vi "stream_only_test.vi"() -> ()   [LabVIEW 2025, in "LabJackEKG.lvlib"]
uses:
  LabJackEKG.lvlib
  <vilib>/Analysis/NI_AALPro.lvlib
panel:
  in  "Sampling Frequency [Hz]":dbl=2500.0
  out "stop":bool
  in  "Samples":i64
  in  "Window":bool
  in  "milliseconds to wait":u32=100
  out "size(s)":i32
  out "Waveform Chart":cluster{dbl, dbl}(graph)
  in  "Number of Stickers":i64
  in  "Samping Window [s]":dbl
  out "error out":errorcluster
  in  "stop":bool
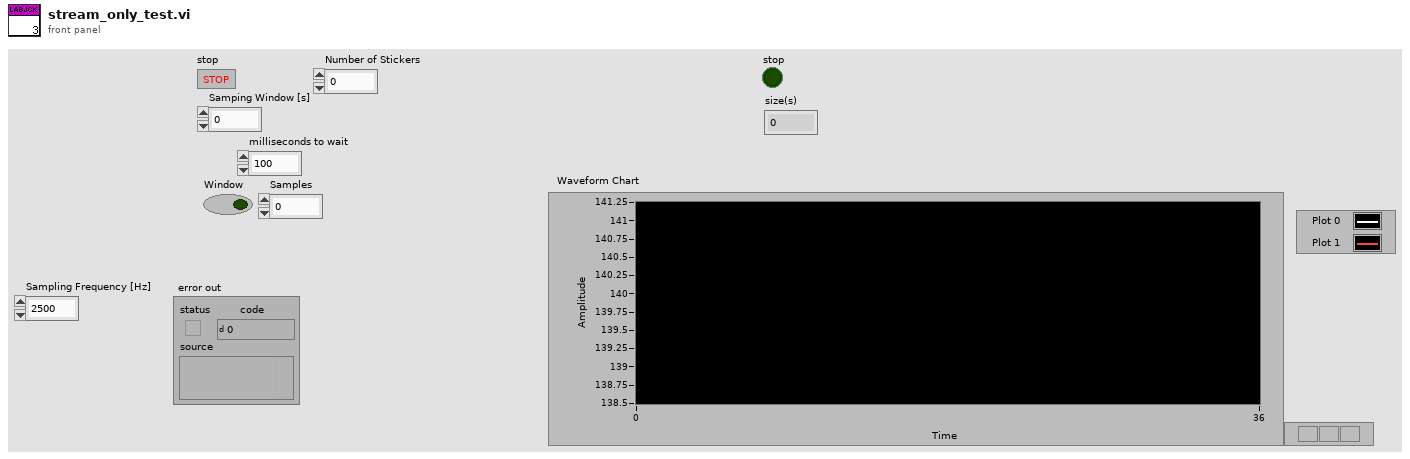
[diagram p1: front panel]
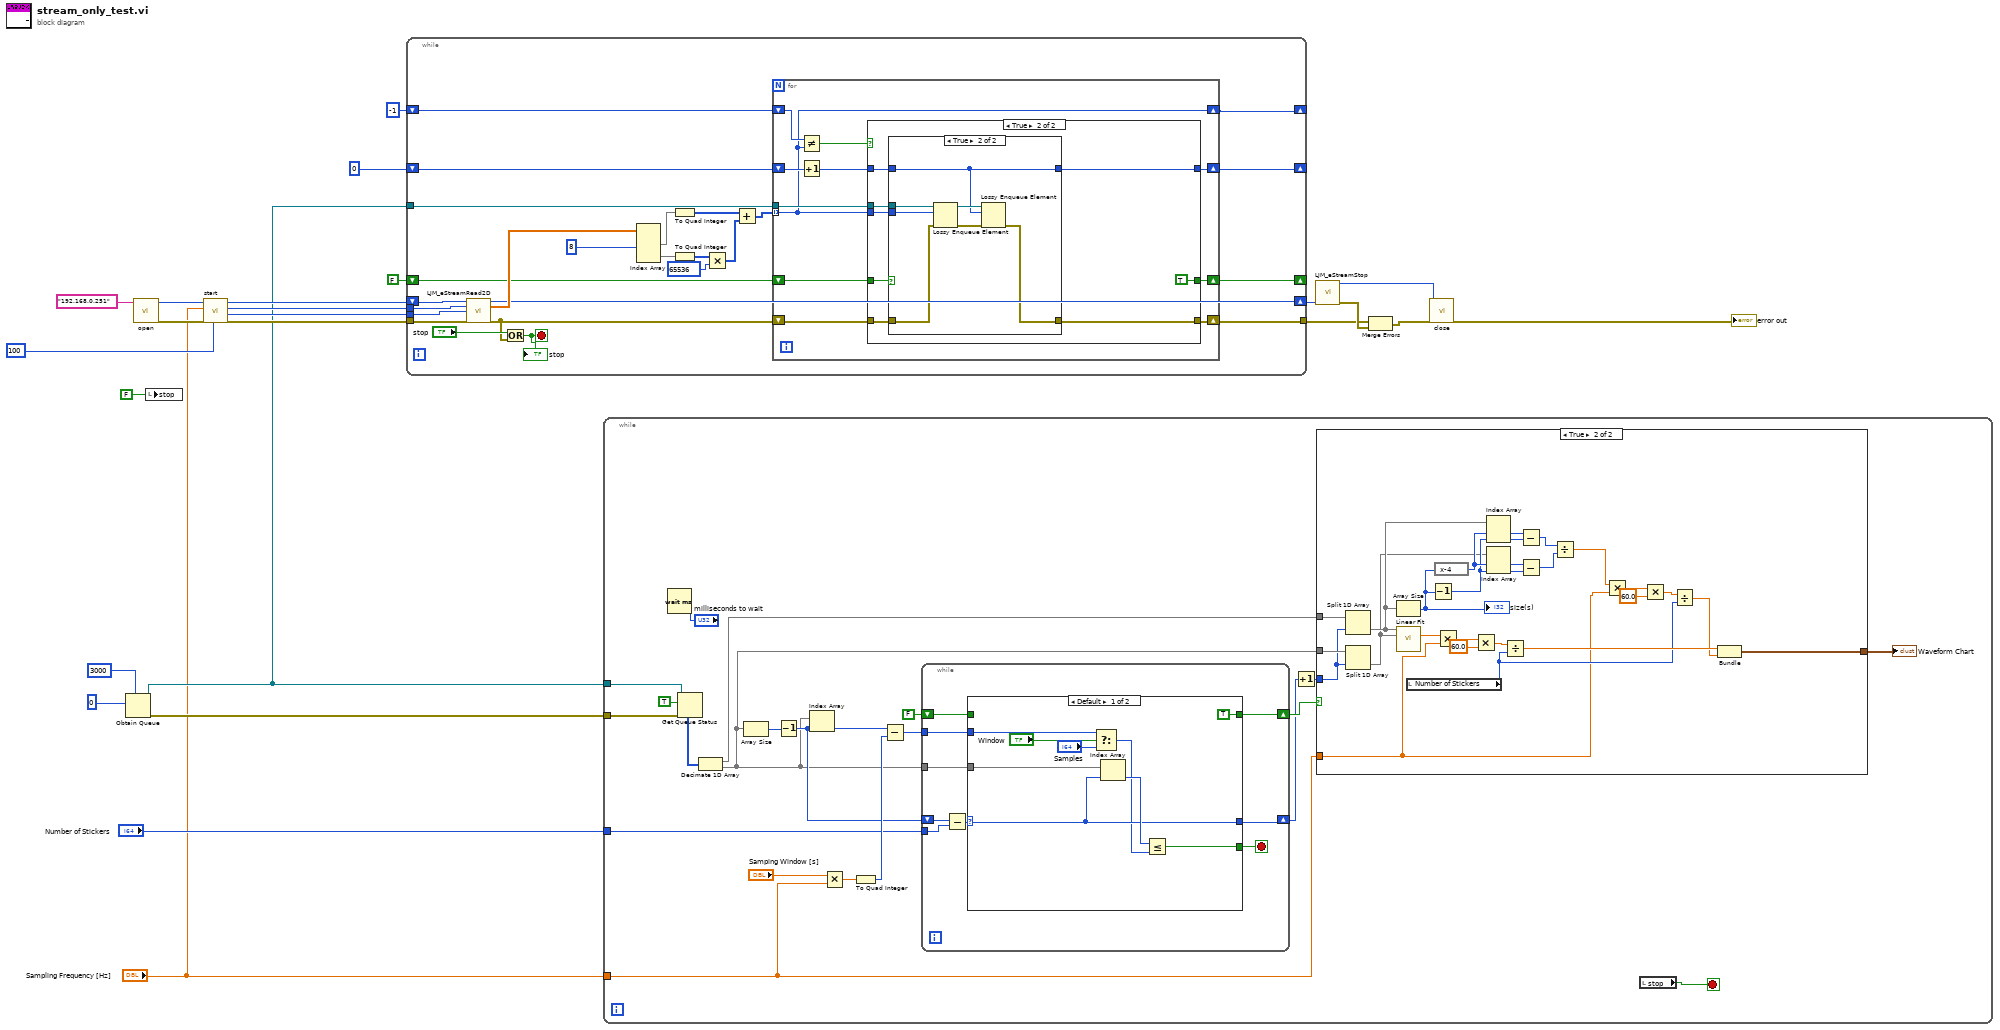
[diagram p0: block diagram]
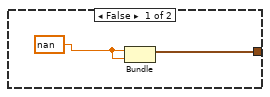
[diagram p4: hidden frame]
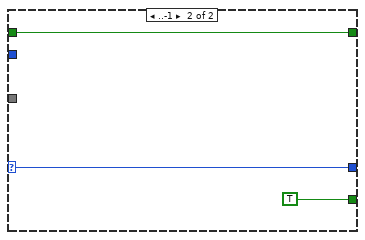
[diagram p5: hidden frame]
diagram:
  n1 = Obtain Queue(max queue size (-1, unlimited)=3000, element data type=i64 0) -> (queue out=w12:refnum<queue>, error out=w14:errorcluster)  [unwired: 3 in, 1 out]
  n2 = call "open.vi"("IP Address (LJM_idANY )"="192.168.0.251") -> ("error out"=w24:errorcluster, "Handle"=w23:i32)  [unwired: 8 in, 1 out]
  n3 = local write "stop"(FALSE ("x .or. y?")) -> ()
  n4 = call "start.vi"("Period [ms]"=100, "error in (no error)"=w24, "Scan Rate (Hz)"="Sampling Frequency [Hz]", "Handle In"=w23) -> ("error out"=w22:errorcluster, "NumReadAddresses"=w19:i32, "ScansPerRead Out"=w20:i32, "Handle Out"=w21:i32)  [unwired: 4 in]
  n5 = while {
    tunnel: w22 -> [w49]
    tunnel: [w38] -> w3
    tunnel: w20 -> [w47]
    tunnel: w19 -> [w48]
    shift-right: [w43] -> w7
    shift-left: w21 -> [w46]
    tunnel: w12 -> [w40]
    shift-right: [w33] -> _
    shift-left: i64 -1 -> [w34]
    shift-right: [w36] -> _
    shift-left: i64 0 -> [w37]
    shift-right: [w25] -> _
    shift-left: FALSE ("x .or. y?") -> [w26]
    stop <- w32 stop-if-true
    n6 = call <vilib>:"LJM_eStreamRead2D.vi"("Handle In"=w46, "ScansPerRead"=w47, "NumAddresses"=w48, "error in"=w49) -> ("Handle Out"=w43:i32, "aData Out"=w45:dbl[][], "error out"=w39:errorcluster)  [unwired: 7 in, 2 out]
    n7 = Or(x="stop", y=w39) -> (x .or. y?=w32:bool)
    "stop" <- w32
    n8 = Index Array(array=w45, index (col) #1=8 ("disabled index (col)")) -> (element #1=w41:dbl[], element #2=w31:dbl[])  [unwired: 3 in]
    n9 = To Quad Integer(1:w41) -> (0:w35:i64[])
    n10 = To Quad Integer(1:w31) -> (0:w30:i64[])
    n11 = Multiply(x=w30, y=i64 65536 ("x")) -> (x*y=w27:i64[])
    n12 = Add(x=w35, y=w27) -> (x+y=w28:i64[])
    n13 = for {
      tunnel: w28 -> [w54] mode=indexing
      tunnel: w40 -> [w60]
      shift-right: [w59] -> w38
      shift-left: w39 -> [w58]
      shift-right: [w57] -> w36
      shift-left: w37 -> [w56]
      shift-right: [w54] -> w33
      shift-left: w34 -> [w55]
      shift-right: [w52] -> w25
      shift-left: w26 -> [w51]
      n14 = Not Equal?(x=w55, y=w54) -> (x != y?=w50:bool)
      n15 = Increment(x=w56) -> (x+1=w53:i64)
      n16 = case shown="True" w50 {
        tunnel: w60 -> [_ w71]
        tunnel: [w63 w68] -> w59
        tunnel: w58 -> [w63 w70]
        tunnel: w54 -> [_ w69]
        tunnel: [w62 w64] -> w57
        tunnel: w53 -> [w62 w67]
        tunnel: [w61 TRUE] -> w52
        tunnel: w51 -> [w61 w65]
        frame False {
        }
        frame True {
          n17 = case shown="True" w65 {
            tunnel: w71 -> [_ w80]
            tunnel: w70 -> [w73 w78]
            tunnel: w69 -> [_ w77]
            tunnel: [w73 w76] -> w68
            tunnel: w67 -> [w72 w74]
            tunnel: [w72 w74] -> w64
            frame False {
            }
            frame True {
              n18 = Lossy Enqueue Element(queue=w80, element=w77, error in (no error)=w78) -> (queue out=w75:refnum<queue>, error out=w79:errorcluster)  [unwired: 2 out]
              n19 = Lossy Enqueue Element(queue=w75, element=w74, error in (no error)=w79) -> (error out=w76:errorcluster)  [unwired: 3 out]
            }
          }
        }
      }
    }
  }
  n20 = while {
    tunnel: w12 -> [w102]
    tunnel: w14 -> [w101]
    tunnel: "Number of Stickers" -> [w94]
    tunnel: "Sampling Frequency [Hz]" -> [w83]
    stop <- w84 stop-if-true
    n21 = Wait (ms)(milliseconds to wait="milliseconds to wait") -> ()  [unwired: 1 out]
    n22 = Get Queue Status(queue=w102, return elements? (F)=TRUE, error in (no error)=w101) -> (elements=w100:i64[])  [unwired: 7 out]
    n23 = Decimate 1D Array(w100) -> (w89:i64[], w82:i64[])
    n24 = Array Size(array=w82) -> (size(s)=w91:i32)
    n25 = Decrement(x=w91) -> (x-1=w90:i32)
    n26 = Index Array(array=w82, index=w90) -> (element=w96:i64)
    n27 = Multiply(x="Samping Window [s]", y=w83) -> (x*y=w99:dbl)
    n28 = To Quad Integer(1:w99) -> (0:w97:i64)
    n29 = Subtract(x=w96, y=w97) -> (x-y=w95:i64)
    n30 = while {
      tunnel: w95 -> [w138]
      shift-right: [w135] -> w86
      shift-left: w90 -> [w132]
      tunnel: w94 -> [w140]
      tunnel: w82 -> [w134]
      shift-right: [w136] -> w88
      shift-left: FALSE -> [w133]
      stop <- w137 stop-if-true
      n31 = Subtract(x=w132, y=w140) -> (x-y=w139:i64)
      n32 = case shown="Default" w139 {
        selector: w139 -> [w145 w151]
        tunnel: w134 -> [w149 _]
        tunnel: w138 -> [w147 _]
        tunnel: [w146 TRUE] -> w137
        tunnel: [TRUE w150] -> w136
        tunnel: [w145 w151] -> w135
        tunnel: w133 -> [_ w150]
        frame Default {
          n33 = Select(t=w147, s="Window", f="Samples") -> (s? t:f=w143:i64)
          n34 = Index Array(array=w149, index=w145) -> (element=w148:i64)
          n35 = Less Or Equal?(x=w148, y=w143) -> (x <= y?=w146:bool)
        }
        frame ..-1 {
        }
      }
    }
    n36 = Increment(x=w86) -> (x+1=w85:i64)
    n37 = case shown="True" w88 {
      tunnel: w82 -> [_ w131]
      tunnel: w89 -> [_ w130]
      tunnel: w85 -> [_ w129]
      tunnel: w83 -> [_ w106]
      tunnel: [w104 w105] -> w81
      frame False {
        w103 = nan
        n38 = Bundle(w103, w103) -> (w104:cluster{dbl, dbl})  [unwired: 1 in]
      }
      frame True {
        n39 = Split 1D Array(array=w130, index=w129) -> (second subarray=w124:i64[])  [unwired: 1 out]
        n40 = Split 1D Array(array=w131, index=w129) -> (second subarray=w107:i64[])  [unwired: 1 out]
        n41 = Array Size(array=w124) -> (size(s)=w109:i32)
        "size(s)" <- w109
        n42 = call <vilib>:"Linear Fit.vi"("Y"=w124, "X"=w107) -> ("slope"=w115:dbl)  [unwired: 9 in, 4 out]
        n43 = local read "Number of Stickers"() -> (w111:i64)
        n44 = Decrement(x=w109) -> (x-1=w122:i32)
        n45 = expression code="x-4"(w109) -> (w123:i32)
        n46 = Multiply(x=w115, y=w106) -> (x*y=w128:dbl)
        n47 = Multiply(x=w128, y=60.0) -> (x*y=w127:dbl)
        n48 = Index Array(array=w124, index #1=w123, index #2=w122) -> (element #1=w119:i64, element #2=w118:i64)
        n49 = Index Array(array=w107, index #1=w123, index #2=w122) -> (element #1=w120:i64, element #2=w121:i64)
        n50 = Divide(x=w127, y=w111) -> (x/y=w125:dbl)
        n51 = Subtract(x=w119, y=w118) -> (x-y=w117:i64)
        n52 = Subtract(x=w120, y=w121) -> (x-y=w116:i64)
        n53 = Divide(x=w117, y=w116) -> (x/y=w108:dbl)
        n54 = Multiply(x=w108, y=w106) -> (x*y=w114:dbl)
        n55 = Multiply(x=w114, y=60.0) -> (x*y=w113:dbl)
        n56 = Divide(x=w113, y=w111) -> (x/y=w110:dbl)
        n57 = Bundle(w125, w110) -> (w105:cluster{dbl, dbl})  [unwired: 1 in]
      }
    }
    "Waveform Chart" <- w81
    n58 = local read "stop"() -> (w84:bool)
  }
  n59 = call <vilib>:"LJM_eStreamStop.vi"("Handle In"=w7) -> ("Handle Out"=w6:i32, "error out"=w4:errorcluster)  [unwired: 13 in]
  n60 = Merge Errors(w3, w4) -> (w5:errorcluster)
  n61 = call "close.vi"("error in"=w5, "Handle"=w6) -> ("error out"=→"error out":errorcluster)  [unwired: 9 in]
